vi "Name Folder Path.vi"(10 "Name":string) -> (2 "Name Folder Path":path)   [LabVIEW 2021, in "_Rename.lvlib" / "_Rename.lvclass"]
uses:
  _Rename.lvclass
  _Rename.lvclass/_Rename.ctl
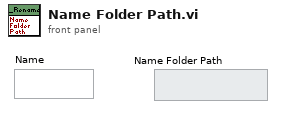
[diagram p1: front panel]
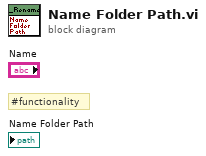
[diagram p0: block diagram]
diagram:
  # "#functionality"
